vi "Log Events.vi"(8 "error in":errorcluster, 10 "Item Names":string[](array[string]), 11 "Event Folder Path":path) -> (0 "error out":errorcluster)   [LabVIEW 2021, in "Game of Life.lvlib"]
doc: "Logs the event record to a CSV file."
uses:
  Game of Life.lvlib
  <vilib>/Utility/file.llb/Write Delimited Spreadsheet (string).vi
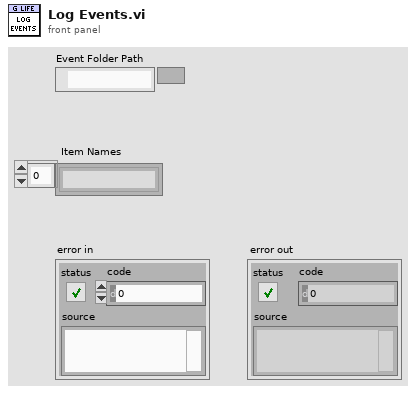
[diagram p1: front panel]
types:
  T1 = enum16{"open", "replace", "create", "open or create", "replace or create", "replace or create with confirmation"}
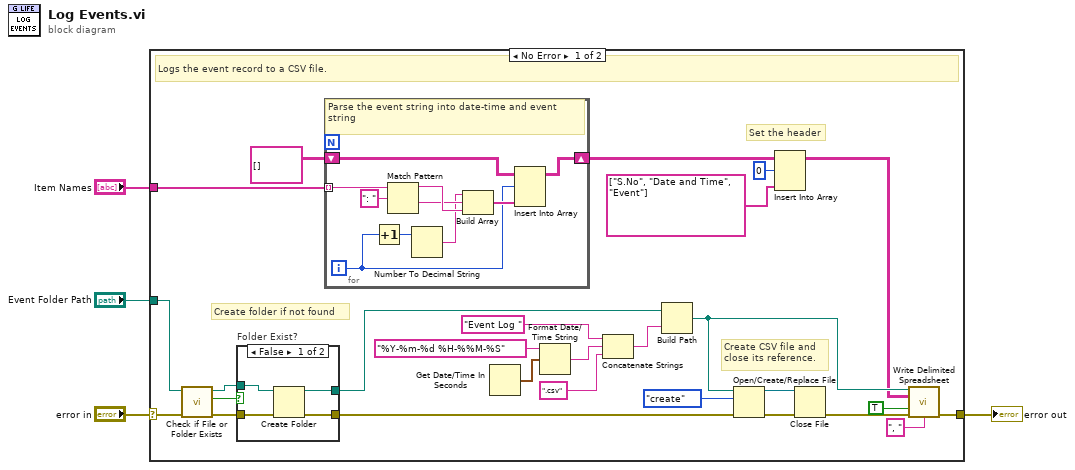
[diagram p0: block diagram]
diagram:
  n1 = case shown="No Error" "error in" {
    selector: "error in" -> [w17 w48]
    tunnel: "Event Folder Path" -> [w18 _]
    tunnel: "Item Names" -> [w26 _]
    tunnel: [w5 w48] -> w1
    frame No Error {
      # "Create CSV file and \nclose its reference."
      # "Create folder if not found"
      # "Set the header"
      # "Logs the event record to a CSV file."
      n2 = call <vilib>:"Check if File or Folder Exists.vi"("error in (no error)"=w17, "path"=w18) -> ("error out"=w15:errorcluster, "file or folder exists?"=w16:bool, "dup path"=w14:path)  [unwired: 7 in]
      n3 = case "Folder Exist?" shown="False" w16 {
        tunnel: w15 -> [w35 w37]
        tunnel: [w34 w37] -> w12
        tunnel: w14 -> [w33 w36]
        tunnel: [w32 w36] -> w13
        frame False {
          n4 = Create Folder(path (use dialog)=w33, error in=w35) -> (created path=w32:path, error out=w34:errorcluster)  [unwired: 1 in, 1 out]
        }
        frame True {
        }
      }
      n5 = for {
        tunnel: w26 -> [w47] mode=indexing
        shift-right: [w41] -> w9
        shift-left: string[][] [] ("Item Names") -> [w42]
        i -> [w40]
        # "Parse the event string into date-time and event string"
        n6 = Increment(x=w40) -> (x+1=w39:i32)
        n7 = Match Pattern(string=w47, regular expression=": ") -> (before substring=w45:string, after substring=w44:string)  [unwired: 1 in, 2 out]
        n8 = Number To Decimal String(number=w39) -> (decimal integer string=w38:string)  [unwired: 1 in]
        n9 = Build Array(w38, w44, w45) -> (w43:string[])
        n10 = Insert Into Array(array=w42, index (row)=w40, new element=w43) -> (w41:string[][])  [unwired: 1 in]
      }
      n11 = Get Date/Time In Seconds() -> (seconds since 1Jan1904=w28:timestamp)
      n12 = Format Date/Time String(time format string (%c)="%Y-%m-%d %H-%%M-%S", seconds (now)=w28) -> (date/time string=w30:string)  [unwired: 1 in]
      n13 = Concatenate Strings("Event Log " ("string"), w30, ".csv" ("string")) -> (w29:string)
      n14 = Build Path(base path=w13, name or relative path=w29) -> (appended path=w21:path)
      n15 = Open/Create/Replace File(file path (use dialog)=w21, error in=w12, operation (0:open)=T1."create") -> (refnum out=w22:refnum<file>, error out=w24:errorcluster)  [unwired: 3 in, 1 out]
      n16 = Insert Into Array(array=w9, index (row)=0, new element=string[] ["S.No", "Date and Time", "Event"] ("new element/subarray")) -> (w8:string[][])  [unwired: 1 in]
      n17 = Close File(refnum=w22, error in=w24) -> (error out=w23:errorcluster)  [unwired: 1 out]
      n18 = call-poly <vilib>:"Write Delimited Spreadsheet.vi"("file path (dialog if empty)"=w21, "2D data"=w8, "append to file? (new file:F)"=TRUE, "error in (no error)"=w23, "delimiter (\\t)"=", " ("delimiter (\\t)")) -> ("error out"=w5:errorcluster)  [unwired: 9 in, 1 out]
    }
    frame Error {
    }
  }
  "error out" <- w1
